vi "GET File Name.vi"() -> (0 "File Name":string)   [LabVIEW 2013]
uses:
  Action.ctl
  Persistent Data FGV Selector.ctl
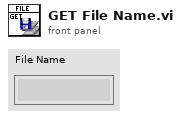
[diagram p1: front panel]
types:
  T1 = typedef "Persistent Data FGV Selector.ctl" = enum16{"Save Directory", "File Name"}
  T2 = typedef "Action.ctl" = enum16{"GET", "PUT", "DELETE"}
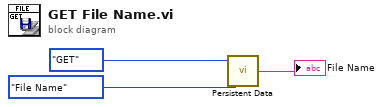
[diagram p0: block diagram]
diagram:
  n1 = call "Persistent Data.vi"("Persistent Data FGV Selector"=Persistent_Data_FGV_Selector."File Name", "Action"=Action."GET") -> ("Output"=→"File Name":string)  [unwired: 1 in]
